vi "File Name to Width_Height.vi"(11 "file name (with xml extension)":string) -> (0 "valid file name?":bool, 1 "keyword":string, 2 "size":T1, 3 "VI file name (no extension)":string)   [LabVIEW 2010, in "NI_SE_Front Panel Layout.lvlib"]
uses:
  NI_SE_Front Panel Layout.lvlib
  <vilib>/Utility/miscctls.llb/LVPointTypeDef.ctl
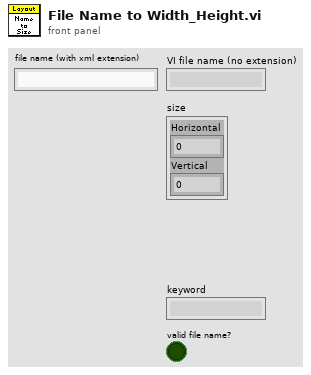
[diagram p1: front panel]
types:
  T1 = typedef "LVPointTypeDef.ctl" = cluster{"Horizontal":i16, "Vertical":i16}
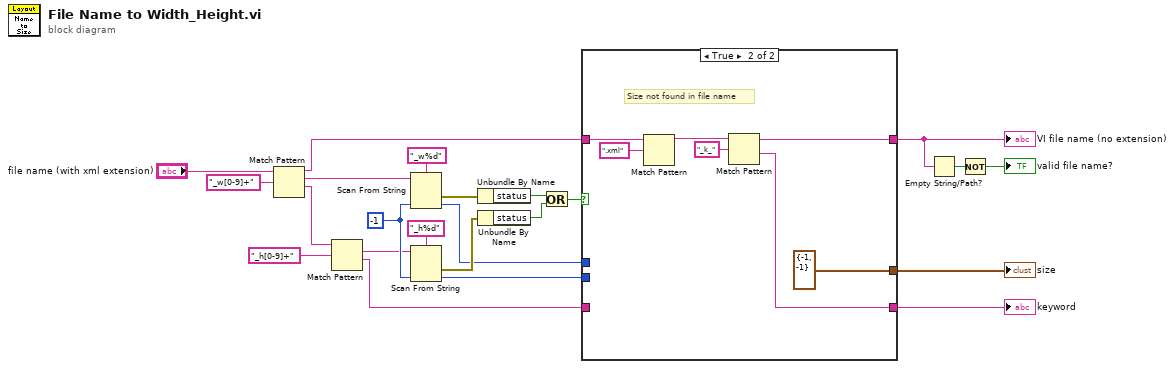
[diagram p0: block diagram]
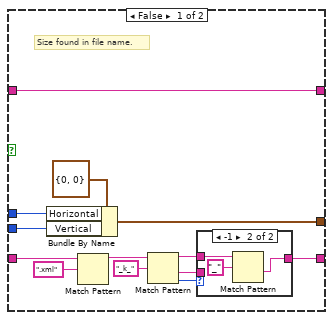
[diagram p2: hidden frame]
diagram:
  w20 = i16 -1 ("default value 1")
  n1 = Match Pattern(string="file name (with xml extension)", regular expression="_w[0-9]+") -> (before substring=w10:string, match substring=w17:string, after substring=w23:string)  [unwired: 1 in, 1 out]
  n2 = Match Pattern(string=w23, regular expression="_h[0-9]+") -> (match substring=w18:string, after substring=w9:string)  [unwired: 1 in, 2 out]
  n3 = Scan From String(format string="_w%d", input string=w17, default 1=w20) -> (error out=w15:errorcluster, output 1=w3:i16)  [unwired: 2 in, 2 out]
  n4 = Scan From String(format string="_h%d", input string=w18, default 1=w20) -> (error out=w14:errorcluster, output 1=w4:i16)  [unwired: 2 in, 2 out]
  n5 = Unbundle By Name(w15) -> ("status"=w13:bool)
  n6 = Unbundle By Name(w14) -> ("status"=w12:bool)
  n7 = Or(x=w13, y=w12) -> (x .or. y?=w11:bool)
  n8 = case shown="True" w11 {
    tunnel: w10 -> [w36 w42]
    tunnel: w9 -> [w28 _]
    tunnel: [w24 w43] -> w1
    tunnel: [w36 w44] -> w7
    tunnel: w4 -> [w33 _]
    tunnel: w3 -> [w34 _]
    tunnel: [w32 T1 {"Horizontal"=-1, "Vertical"=-1} ("size")] -> w2
    frame False {
      # "Size found in file name."
      n9 = Bundle By Name(cluster=T1 {"Horizontal"=0, "Vertical"=0} ("size"), "Horizontal"=w34, "Vertical"=w33) -> (w32:T1)
      n10 = Match Pattern(string=w28, regular expression=".xml") -> (before substring=w30:string)  [unwired: 1 in, 3 out]
      n11 = Match Pattern(string=w30, regular expression="_k_") -> (before substring=w25:string, after substring=w26:string, offset past match=w27:i32)  [unwired: 1 in, 1 out]
      n12 = case shown="-1" w27 {
        tunnel: w26 -> [w37 _]
        tunnel: w25 -> [_ w40]
        tunnel: [w37 w38] -> w24
        frame Default {
        }
        frame -1 {
          n13 = Match Pattern(string=w40, regular expression="_") -> (after substring=w38:string)  [unwired: 1 in, 3 out]
        }
      }
    }
    frame True {
      # "Size not found in file name"
      n14 = Match Pattern(string=w42, regular expression=".xml") -> (before substring=w46:string)  [unwired: 1 in, 3 out]
      n15 = Match Pattern(string=w46, regular expression="_k_") -> (before substring=w44:string, after substring=w43:string)  [unwired: 1 in, 2 out]
    }
  }
  "keyword" <- w1
  "VI file name (no extension)" <- w7
  "size" <- w2
  n16 = Empty String/Path?(string/path=w7) -> (empty?=w6:bool)
  n17 = Not(x=w6) -> (.not. x?=→"valid file name?":bool)
